vi "Calibrate Ticks 2 RT Parameters (uSMC).vi"(2 "RTMinError (ticks)":u16, 3 "RTDelta (ticks)":u16) -> (0 "RTMinError (a.u.)":u16, 1 "RTDelta (a.u.)":u16)   [LabVIEW 2010, in "SignalWriterMH110203USBStepperMotor.lvclass"]
uses:
  SignalWriterMH110203USBStepperMotor.lvclass
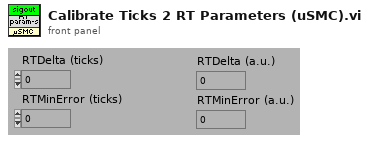
[diagram p1: front panel]
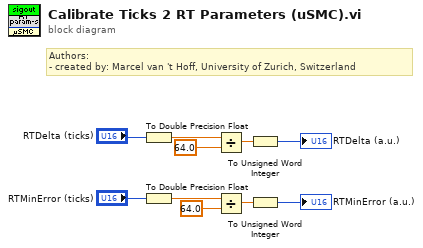
[diagram p0: block diagram]
diagram:
  # "Authors: \n- created by: Marcel van 't Hoff, University of Zurich, Switzerland"
  n1 = To Double Precision Float(number="RTDelta (ticks)") -> (double precision float=w1:dbl)
  n2 = To Double Precision Float(number="RTMinError (ticks)") -> (double precision float=w2:dbl)
  n3 = Divide(x=w1, y=64.0) -> (x/y=w8:dbl)
  n4 = Divide(x=w2, y=64.0) -> (x/y=w6:dbl)
  n5 = To Unsigned Word Integer(number=w8) -> (unsigned 16bit integer=→"RTDelta (a.u.)":u16)
  n6 = To Unsigned Word Integer(number=w6) -> (unsigned 16bit integer=→"RTMinError (a.u.)":u16)
